vi "Bit Manipulation.Set Bit (U16).vi"(9 "bit index":i32, 10 "bit":bool, 11 "packed value in":u16 format="%016x") -> (3 "packed value out":u16 format="%016x")   [LabVIEW 2016, in "VeriStand Data.lvlib"]
doc: "This VI overwrites the bit located at <B>bit index</B> in <B>packed value</B> with the provided <B>bit</B>."
uses:
  VeriStand Data.lvlib
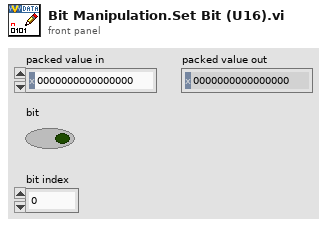
[diagram p1: front panel]
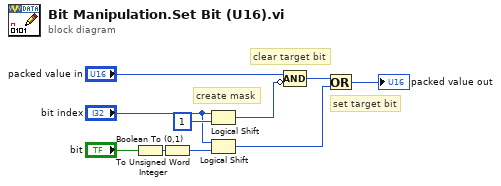
[diagram p0: block diagram]
diagram:
  # "set target bit"
  # "create mask"
  # "clear target bit"
  n1 = Boolean To (0,1)(Boolean="bit") -> (0, 1=w6:i16)
  n2 = To Unsigned Word Integer(number=w6) -> (unsigned 16bit integer=w4:u16)
  n3 = Logical Shift(y="bit index", x=u16 1) -> (x << y=w2:u16)
  n4 = Logical Shift(y="bit index", x=w4) -> (x << y=w5:u16)
  n5 = Compound Arithmetic op=AND("packed value in", invert w2) -> (w8:u16)
  n6 = Or(x=w8, y=w5) -> (x .or. y?=→"packed value out":u16)
